vi "GetSampleData.vi"(8 "错误输入（无错误）":errorcluster, 11 "SampleInfoTime":string) -> (0 "错误输出":errorcluster, 1 "是否存在记录":bool, 2 "记录数":i32, 3 "所有记录":string[][](array[string]))   [LabVIEW 2014, in "cyy.lvlib"]
uses:
  CYY/cyy.lvlib
  DataBase.lvlib
  DetectElecrodes/DetectElectros.lvlib
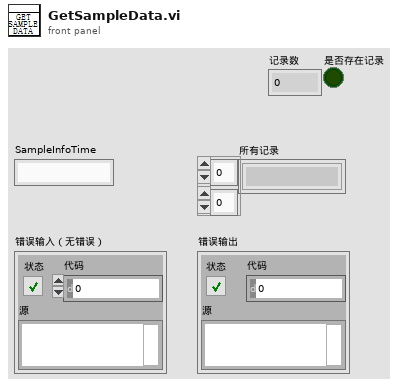
[diagram p1: front panel]
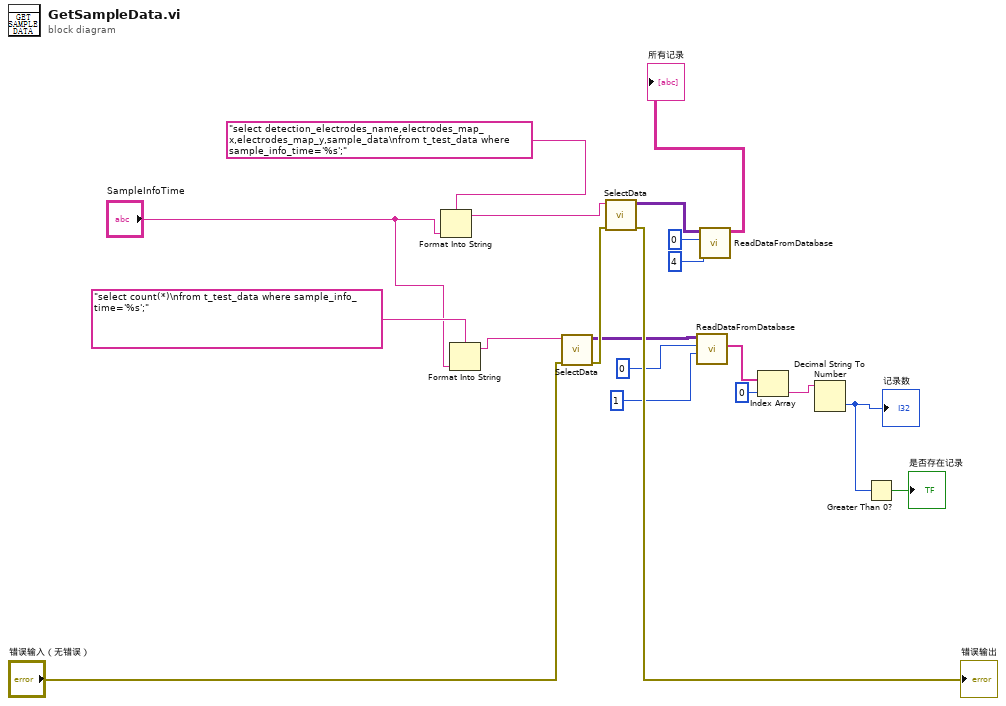
[diagram p0: block diagram]
diagram:
  n1 = Format Into String(format string="select detection_electrodes_name,electrodes_map_x,electrodes_map_y,sample_data\nfrom t_test_data where sample_info_time='%s';", "SampleInfoTime") -> (resulting string=w14:string)  [unwired: 2 in, 1 out]
  n2 = Format Into String(format string="select count(*)\nfrom t_test_data where sample_info_time='%s';", "SampleInfoTime") -> (resulting string=w11:string)  [unwired: 2 in, 1 out]
  n3 = call "SelectData.vi"("SQL query"=w11, "error in"="错误输入（无错误）") -> ("recordset data"=w8:variant[][], "error out"=w10:errorcluster)  [unwired: 6 in]
  n4 = call "SelectData.vi"("SQL query"=w14, "error in"=w10) -> ("recordset data"=w17:variant[][], "error out"=→"错误输出":errorcluster)  [unwired: 6 in]
  n5 = call "ReadDataFromDatabase.vi"("长度"=1, "index"=0, "recordset data"=w8) -> ("一行记录"=w5:string[])  [unwired: 7 in, 1 out]
  n6 = call "ReadDataFromDatabase.vi"("长度"=4, "index"=0, "recordset data"=w17) -> ("所有记录"=→"所有记录":string[][])  [unwired: 7 in, 1 out]
  n7 = Index Array(array=w5, index=0 ("索引")) -> (element=w3:string)
  n8 = Decimal String To Number(string=w3) -> (number=w2:i32)  [unwired: 2 in, 1 out]
  "记录数" <- w2
  n9 = Greater Than 0?(x=w2) -> (x > 0?=→"是否存在记录":bool)
